vi "Unique_D.vi"(11 "1D Array In":dbl[](array[numeric])=[1.0, -1.0, 3.0, 8.0, 3.0]) -> (3 "Boolean":bool)   [LabVIEW 2013]
doc: "Returns whether the array consists of unique values without repetition."
uses:
  UniqueLast_D.vi
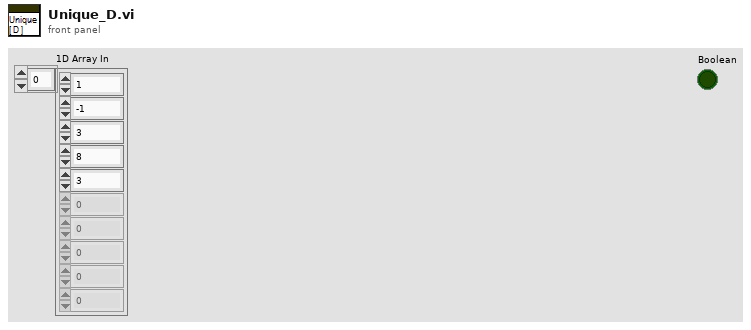
[diagram p1: front panel]
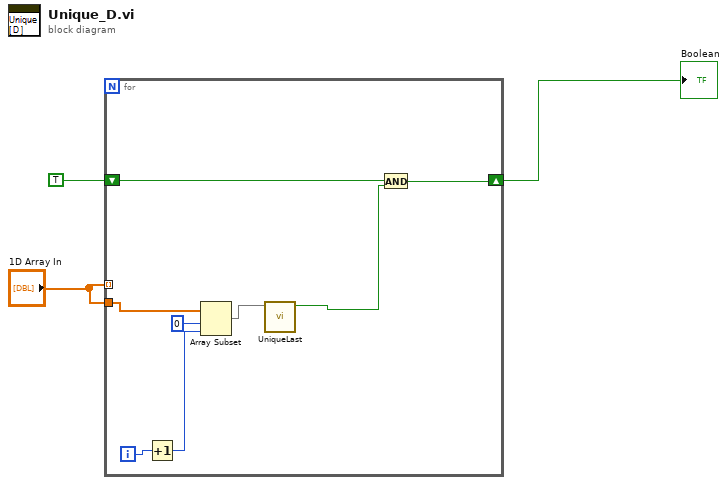
[diagram p0: block diagram]
diagram:
  n1 = for {
    shift-right: [w9] -> w2
    shift-left: TRUE -> [w8]
    tunnel: "1D Array In" -> [w7]
    tunnel: "1D Array In" -> [_] mode=indexing
    i -> [w11]
    n2 = Increment(x=w11) -> (x+1=w10:i32)
    n3 = Array Subset(array=w7, index=0, length=w10) -> (w6:dbl[])
    n4 = call-poly "UniqueLast.vi"("1D Array In"=w6) -> ("Boolean"=w5:bool)  [unwired: 10 in]
    n5 = And(x=w8, y=w5) -> (x .and. y?=w9:bool)
  }
  "Boolean" <- w2
